vi "Create XML Editor.vi"(8 "error in (no error)":errorcluster, 10 "XML or Project Path":path) -> (0 "error out":errorcluster, 3 "Project XML Editor out":refnum<class "Project XML Editor.lvclass">)   [LabVIEW 2018, in ".LVLIBP CD XML Updater.lvlib" / "Project XML Editor.lvclass"]
uses:
  Project XML Editor.lvclass
  Project XML Editor.lvclass/Project XML Editor.ctl
  <vilib>/xml/Load XML File.vi
  <vilib>/xml/NI_XML.lvlib
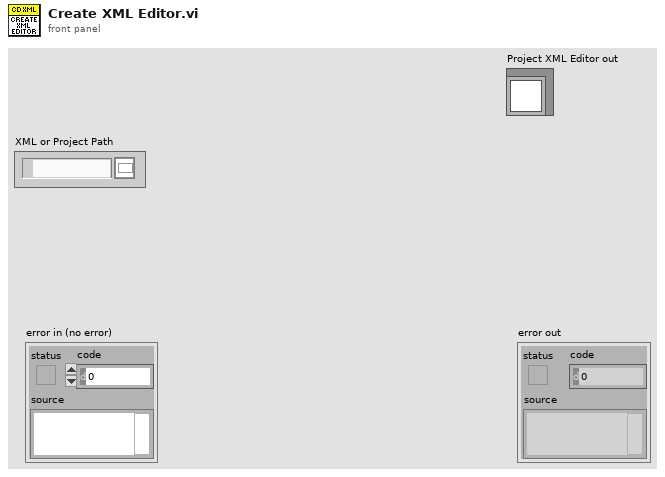
[diagram p1: front panel]
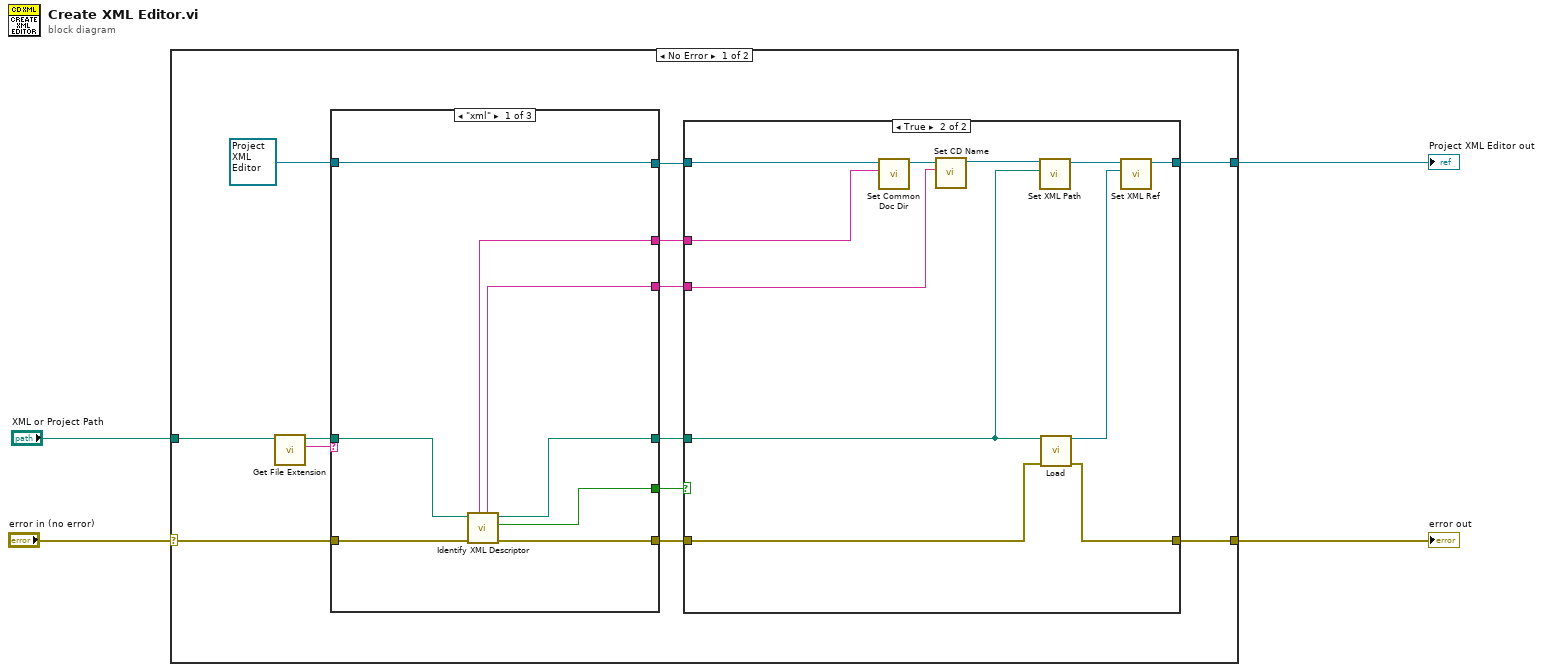
[diagram p0: block diagram]
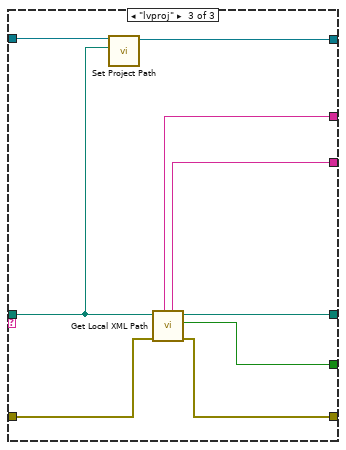
[diagram p4: hidden frame]
diagram:
  n1 = case shown="No Error" "error in (no error)" {
    selector: "error in (no error)" -> [w17 w51]
    tunnel: [w13 w51] -> w3
    tunnel: [w12 _] -> w2
    tunnel: "XML or Project Path" -> [w9 _]
    frame No Error {
      n2 = call <vilib>:"Get File Extension.vi"("file"=w9) -> ("lowercase file extension"=w8:string, "dup file"=w7:path)  [unwired: 6 in, 3 out]
      n3 = case shown="\"xml\"" w8 {
        tunnel: w17 -> [w38 w41 w50]
        tunnel: [w35 w41 w49] -> w16
        tunnel: [w36 w39 w48] -> w14
        tunnel: [w34 _ w47] -> w15
        tunnel: [w32 _ w46] -> w11
        tunnel: [w33 _ w45] -> w10
        tunnel: w7 -> [w37 w39 w43]
        tunnel: refnum<class "Project XML Editor.lvclass"> refnum ("Project XML Editor in") -> [w31 w40 w44]
        tunnel: [w31 w40 w42] -> w5
        frame "xml" {
          n4 = call "Identify XML Descriptor.vi"("error in"=w38, "XML Path in"=w37) -> ("error out"=w35:errorcluster, "Found ?"=w34:bool, "XML Path out"=w36:path, "Custom Device Name"=w33:string, "Common Doc Dir"=w32:string)  [unwired: 5 in]
        }
        frame "None", Default {
        }
        frame "lvproj" {
          n5 = call "Set Project Path.vi"("Source Project Path"=w43, "Project XML Editor in"=w44) -> ("Project XML Editor out"=w42:refnum<class "Project XML Editor.lvclass">)  [unwired: 9 in]
          n6 = call "Get Local XML Path.vi"("Error In"=w50, "Project Path"=w43) -> ("Error Out"=w49:errorcluster, "Found ?"=w47:bool, "XML Path"=w48:path, "Custom Device Name"=w45:string, "Common Doc Dir"=w46:string)  [unwired: 5 in]
        }
      }
      n7 = case shown="True" w15 {
        tunnel: w16 -> [w19 w30]
        tunnel: w14 -> [_ w27]
        tunnel: [w19 w29] -> w13
        tunnel: w5 -> [w18 w24]
        tunnel: [w18 w25] -> w12
        tunnel: w11 -> [_ w21]
        tunnel: w10 -> [_ w20]
        frame False {
        }
        frame True {
          n8 = call "Set Common Doc Dir.vi"("Common Doc Dir"=w21, "Project XML Editor in"=w24) -> ("Project XML Editor out"=w23:refnum<class "Project XML Editor.lvclass">)  [unwired: 9 in]
          n9 = call "Set CD Name.vi"("CD Name"=w20, "Project XML Editor in"=w23) -> ("Project XML Editor out"=w22:refnum<class "Project XML Editor.lvclass">)  [unwired: 9 in]
          n10 = call "Set XML Path.vi"("XML Path"=w27, "Project XML Editor in"=w22) -> ("Project XML Editor out"=w28:refnum<class "Project XML Editor.lvclass">)  [unwired: 9 in]
          n11 = call-poly <vilib>:"Load.vi"("path to XML document"=w27, "error in (no error)"=w30) -> ("DOM document out"=w26:refnum<k20>, "error out"=w29:errorcluster)  [unwired: 11 in, 1 out]
          n12 = call "Set XML Ref.vi"("XML Ref"=w26, "Project XML Editor in"=w28) -> ("Project XML Editor out"=w25:refnum<class "Project XML Editor.lvclass">)  [unwired: 9 in]
        }
      }
    }
    frame Error {
    }
  }
  "error out" <- w3
  "Project XML Editor out" <- w2
